vi "Get Collection Items.vi"(8 "error in (no error)":errorcluster, 10 "Collection":variant) -> (0 "error out":errorcluster, 2 "Items":variant[](array[variant]))   [LabVIEW 2017, in "Transparent Assertions.lvlib" / "Constraints.lvlib"]
uses:
  Constraints.lvlib
  <vilib>/Utility/error.llb/Error Cluster From Error Code.vi
  <vilib>/ErrorRing/Error Ring.xnode
  <vilib>/PNR/LabVIEW Composition/Composition/Composition.lvlib
  <vilib>/Utility/Data Type/NI_Data Type.lvlib
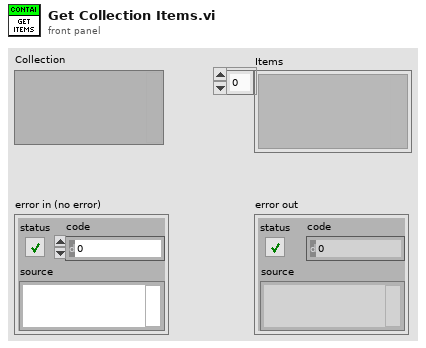
[diagram p1: front panel]
types:
  T1 = typedef "NI_Data Type.lvlib/Data Type.ctl" = enum8{"Invalid Type", "Void", "I8", "I16", "I32", "I64", "U8", "U16", "U32", "U64", "Single Float", "Double Float", "Extended Float", "Single Complex", "Double Complex", "Extended Complex", "Enum U8", "Enum U16", "Enum U32", "Enum U64", "Single Float With Unit", "Double Float With Unit", "Extended Float With Unit", "Single Complex with Unit", "Double Complex with Unit", "Extended Complex with Unit", "Boolean", "String", "Path", "Picture", "Tag", "Array", "Cluster", "Variant", "LV Variant", "Waveform", "Timestamp", "Digital Waveform", "Digital Data", "ExpressData", "Refnum", "External Data", "VI", "Poly VI", "LabVIEW Class Instance", "Fixed Point"}
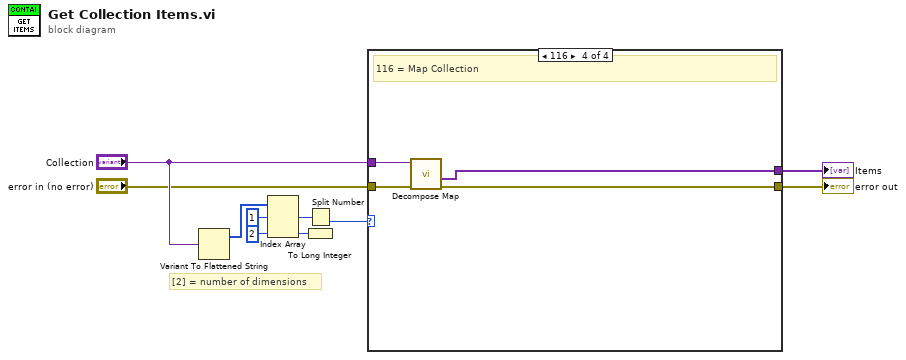
[diagram p0: block diagram]
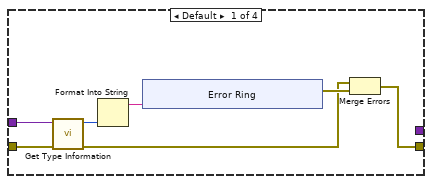
[diagram p2: hidden frame]
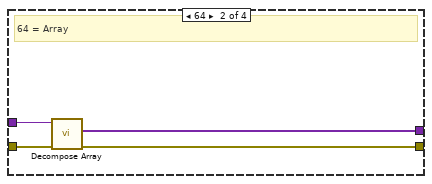
[diagram p3: hidden frame]
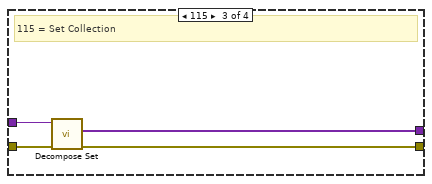
[diagram p4: hidden frame]
diagram:
  # "[2] = number of dimensions"
  n1 = Variant To Flattened String(Variant="Collection") -> (1:w8:i16[])  [unwired: 1 out]
  n2 = Index Array(array=w8, index #1=1 ("index"), index #3=2 ("index")) -> (element #1=w9:i16, element #3=w6:i16)  [unwired: 1 in, 1 out]
  n3 = To Long Integer(number=w6) -> ()  [unwired: 1 out]
  n4 = Split Number(x=w9) -> (lo(x)=w5:u8)  [unwired: 1 out]
  n5 = case shown="116" w5 {
    tunnel: "error in (no error)" -> [w13 w28 w32 w36]
    tunnel: [w11 w27 w31 w35] -> w2
    tunnel: "Collection" -> [w14 w26 w30 w34]
    tunnel: [_ w25 w29 w33] -> w1
    frame Default {
      n6 = call <vilib>:"Get Type Information.vi"("error in (no error)"=w13, "Variant"=w14) -> ("error out"=w12:errorcluster, "Type"=w15:T1)  [unwired: 5 in, 3 out]
      n7 = Format Into String(w15) -> (resulting string=w16:string)  [unwired: 3 in, 1 out]
      n8 = xnode "Error Ring"("parameter 0"=w16) -> ("error out"=w17:errorcluster)
      n9 = Merge Errors(w12, w17) -> (w11:errorcluster)
    }
    frame 64 {
      # "64 = Array"
      n10 = call <vilib>:"Decompose Array.vi"("error in (no error)"=w28, "Variant Array"=w26) -> ("error out"=w27:errorcluster, "Elements"=w25:variant[])  [unwired: 6 in, 2 out]
    }
    frame 115 {
      # "115 = Set Collection"
      n11 = call <vilib>:"Decompose Set.vi"("error in (no error)"=w32, "Variant Set"=w30) -> ("error out"=w31:errorcluster, "Elements"=w29:variant[])  [unwired: 7 in, 1 out]
    }
    frame 116 {
      # "116 = Map Collection"
      n12 = call <vilib>:"Decompose Map.vi"("error in (no error)"=w36, "Variant Map"=w34) -> ("error out"=w35:errorcluster, "Values"=w33:variant[])  [unwired: 6 in, 2 out]
    }
  }
  "error out" <- w2
  "Items" <- w1
